vi "ACK Subscriptions Publications.vi"(0 "GEA2 Reference In":refnum<k24>, 7 "GEA2 Msg":T1 {"Command" format="%02x"; "Destination" format="%02x"; "Source" format="%02x"}, 11 "error in (no error)":errorcluster) -> (4 "GEA2 Reference Out":refnum<k24>, 15 "error out":errorcluster)   [LabVIEW 2023]
uses:
  Common/LabVIEW GEA2 Toolkit/GEA3/type defs/Data In.ctl
  D:/Common/LabVIEW GEA2 Toolkit/source/GEA3 DLL Source/GeaCommunication.dll
  Common/LabVIEW GEA2 Toolkit/source/GEA3 DLL Source/GeaCommunication.dll
  Common/LabVIEW GEA2 Toolkit/GEA3/library/GEA2_Toolkit.lvlib
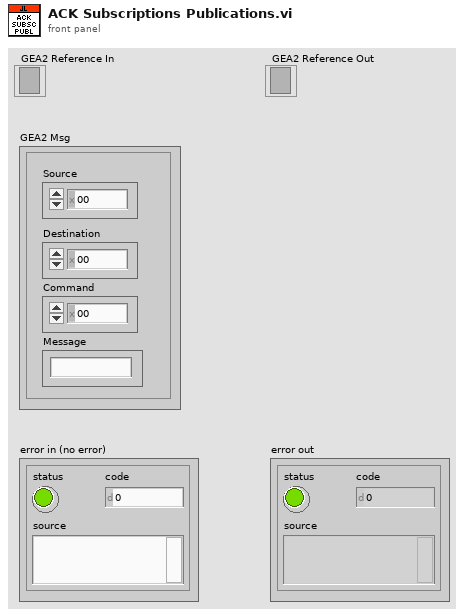
[diagram p1: front panel]
types:
  T1 = typedef "Data In.ctl" = cluster{"Source":u8, "Destination":u8, "Command":u8, "Message":string}
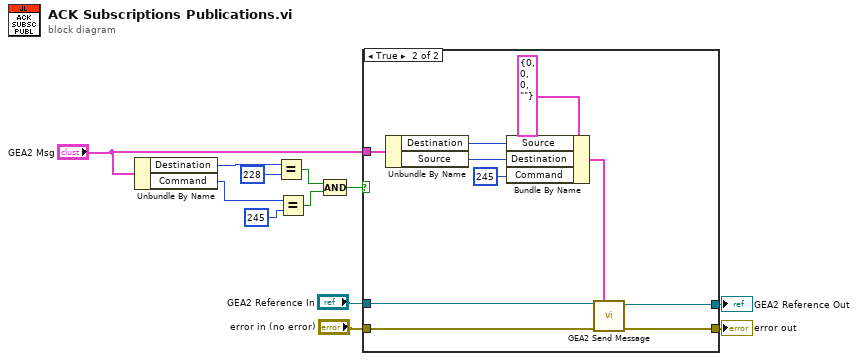
[diagram p0: block diagram]
diagram:
  n1 = Unbundle By Name("GEA2 Msg") -> ("Destination"=w8:u8, "Command"=w5:u8)
  n2 = Equal?(x=w8, y=u8 228) -> (x = y?=w7:bool)
  n3 = Equal?(x=w5, y=u8 245) -> (x = y?=w3:bool)
  n4 = Compound Arithmetic op=AND(w7, w3) -> (w12:bool)
  n5 = case shown="True" w12 {
    tunnel: "error in (no error)" -> [w14 w24]
    tunnel: [w14 w15] -> w11
    tunnel: "GEA2 Msg" -> [_ w23]
    tunnel: "GEA2 Reference In" -> [w13 w18]
    tunnel: [w13 w17] -> w1
    frame False {
    }
    frame True {
      n6 = Unbundle By Name(w23) -> ("Destination"=w19:u8, "Source"=w21:u8)
      n7 = Bundle By Name(cluster=T1 {"Source"=0, "Destination"=0, "Command"=0, "Message"=""} ("GEA2 Msg"), "Source"=w19, "Destination"=w21, "Command"=u8 245) -> (w16:T1)
      n8 = call "GEA2 Send Message.vi"("GEA2 Reference In"=w18, "Input Data"=w16, "Error In"=w24) -> ("GEA2 Reference Out"=w17:refnum<k24>, "Error Out"=w15:errorcluster)  [unwired: 11 in]
    }
  }
  "error out" <- w11
  "GEA2 Reference Out" <- w1
